vi "Configure Voltage Level.vi"(7 "Mode":T2 items=["AC", "DC", "IR"], 8 "error in (no error)":errorcluster, 9 "Voltage Level [V]":u16=1000 min=50 max=6000 step=1 format="%.3p", 10 "Step":T1=1 min=1 max=99 step=1, 11 "VISA resource name":refnum<visa-resource-name>) -> (0 "error out":errorcluster, 3 "VISA resource name out":refnum<visa-resource-name>)   [LabVIEW 2025]
uses:
  <instrlib>/Chrome 19025/Public/Utility/Type Def/AC-DC-IR modes--ring.ctl
  <instrlib>/Chrome 19025/Public/Utility/Type Def/steps--numeric.ctl
panel:
  # "Set Voltage Level"
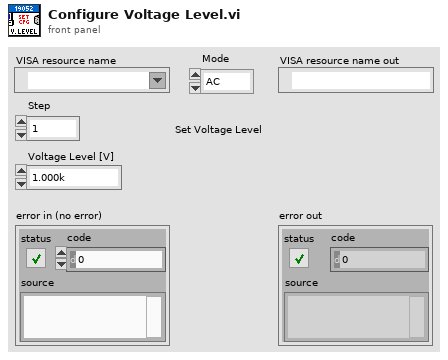
[diagram p1: front panel]
types:
  T1 = typedef "Chrome 19025.lvlib/steps--numeric.ctl" = u8
  T2 = typedef "Chrome 19025.lvlib/AC-DC-IR modes--ring.ctl" = u16
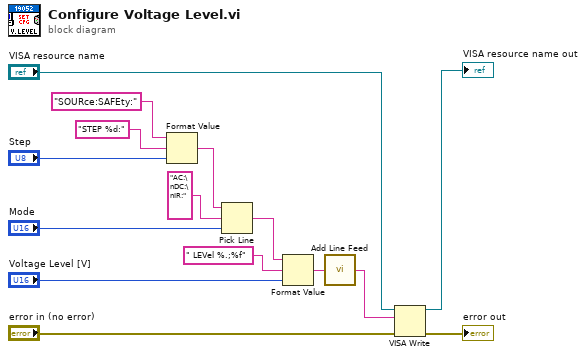
[diagram p0: block diagram]
diagram:
  n1 = Format Value(string ("")="SOURce:SAFEty:", format string="STEP %d:", value (0)="Step") -> (output string=w8:string)
  n2 = Pick Line(string ("")=w8, multi-line string="AC:\nDC:\nIR:", line index="Mode") -> (output string=w7:string)
  n3 = Format Value(string ("")=w7, format string=" LEVel %.;%f", value (0)="Voltage Level [V]") -> (output string=w6:string)
  n4 = call <instrlib>:"Add Line Feed.vi"("Command string"=w6) -> ("Concatenated string"=w5:string)  [unwired: 4 in]
  n5 = VISA Write(VISA resource name="VISA resource name", write buffer=w5, error in (no error)="error in (no error)") -> (VISA resource name out=→"VISA resource name out":refnum<visa-resource-name>, error out=→"error out":errorcluster)  [unwired: 1 out]
